vi "PID_ini.vi"(8 "Enable_sat":bool=TRUE, 9 "T_control":enum16{"Manifold", "Bobina"}(ring)=enum."Bobina", 10 "Saturacion_manifold":dbl=92.0, 11 "PID gains":T1) -> (3 "PID_Bitron out":refnum<class "PID_Bitron.lvclass">)   [LabVIEW 2022 SP3, in "PID_Bitron.lvclass"]
uses:
  PID_Bitron.lvclass
  PID_Bitron.lvclass/PID_Bitron.ctl
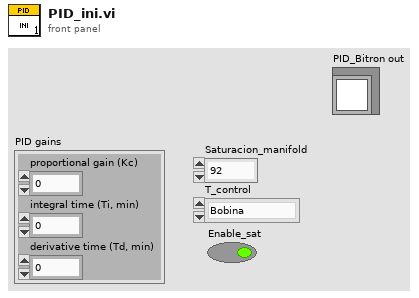
[diagram p1: front panel]
types:
  T1 = cluster{"proportional gain (Kc)":dbl, "integral time (Ti, min)":dbl, "derivative time (Td, min)":dbl}
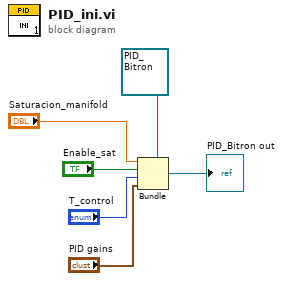
[diagram p0: block diagram]
diagram:
  n1 = Bundle(cluster=refnum<class "PID_Bitron.lvclass"> refnum ("PID_Bitron.lvclass 2"), "Saturacion_manifold", "Enable_sat", "T_control", "PID gains") -> (→"PID_Bitron out":refnum<class "PID_Bitron.lvclass">)
